vi "Write to Motor State.vi"(8 "error in (no error)":errorcluster, 9 "state mode":T1 items=["undefined", "angle", "velocity"], 10 "value":dbl, 11 "motor state in":T2={"angle"=0.0, "velocity"=0.0, "state mode"=1} {"state mode" items=["undefined", "angle", "velocity"]}) -> (0 "error out":errorcluster, 1 "failed?":bool, 3 "motor state out":T2={"angle"=0.0, "velocity"=0.0, "state mode"=1} {"state mode" items=["undefined", "angle", "velocity"]})   [LabVIEW 2017, in "NI_Robotics_Motor Communication.lvclass"]
uses:
  <vilib>/robotics/Actuation/Motor Communication/NI_Robotics_Motor Communication.lvclass
  <vilib>/robotics/Actuation/Motor Communication/Motor State Value.ctl
  <vilib>/robotics/Actuation/Motor Communication/Motor State Mode.ctl
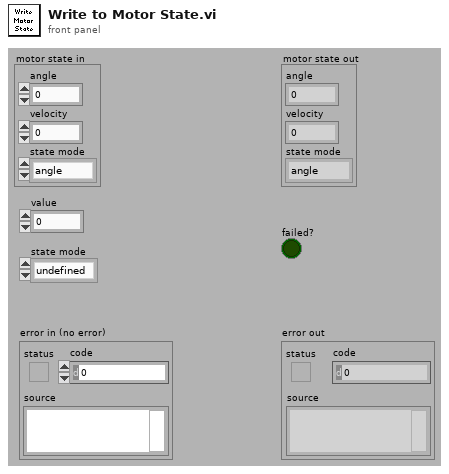
[diagram p1: front panel]
types:
  T1 = typedef "NI_Robotics_Motor Communication.lvclass/Motor State Mode.ctl" = u16
  T2 = typedef "NI_Robotics_Motor Communication.lvclass/Motor State Value.ctl" = cluster{"angle":dbl, "velocity":dbl, "state mode":T1}
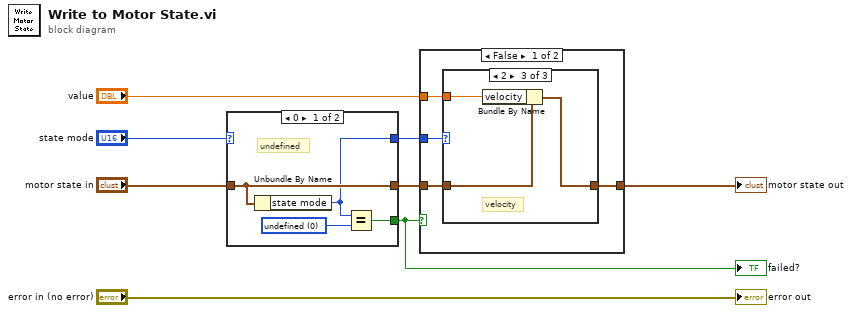
[diagram p0: block diagram]
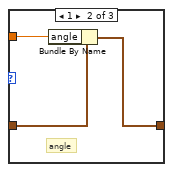
[diagram p3: hidden frame]
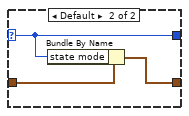
[diagram p5: hidden frame]
diagram:
  n1 = case shown="0" "state mode" {
    selector: "state mode" -> [_ w13]
    tunnel: "motor state in" -> [w12 w15]
    tunnel: [w12 w14] -> w2
    tunnel: [w10 w13] -> w1
    tunnel: [w9 _] -> w3
    frame 0 {
      w11 = T1 0 items=["undefined", "angle", "velocity"] ("state mode")
      # "undefined"
      n2 = Unbundle By Name(w12) -> ("state mode"=w10:T1)
      n3 = Equal?(x=w10, y=w11) -> (x = y?=w9:bool)
    }
    frame Default {
      n4 = Bundle By Name(cluster=w15, "state mode"=w13) -> (w14:T2)
    }
  }
  "failed?" <- w3
  n5 = case shown="False" w3 {
    tunnel: "value" -> [w19 _]
    tunnel: [w18 w27] -> w7
    tunnel: w2 -> [w17 w27]
    tunnel: w1 -> [w16 _]
    frame False {
      n6 = case shown="2" w16 {
        tunnel: w19 -> [_ w23 w26]
        tunnel: w17 -> [w20 w22 w25]
        tunnel: [w20 w21 w24] -> w18
        frame Default {
        }
        frame 1 {
          # "angle"
          n7 = Bundle By Name(cluster=w22, "angle"=w23) -> (w21:T2)
        }
        frame 2 {
          # "velocity"
          n8 = Bundle By Name(cluster=w25, "velocity"=w26) -> (w24:T2)
        }
      }
    }
    frame True {
    }
  }
  "motor state out" <- w7
  "error out" <- "error in (no error)"
